vi "tiaoshi.vi"   [LabVIEW 2020]
types:
  T1 = enum32{"Invalid", "Standard", "Closed", "Hidden", "Minimized", "Maximized"}
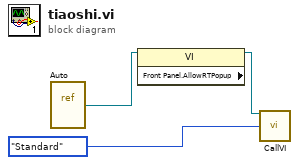
[diagram p0: block diagram]
diagram:
  n1 = vi-ref "Auto.vi"() -> (w2:refnum<vi>)
  n2 = property class="VI" props=["Front Panel.AllowRTPopup"](reference=w2) -> (reference out=w1:refnum<vi>)  [unwired: 1 in, 2 out]
  n3 = call "CallVI.vi"("VI引用"=w1, "状态"=T1."Standard") -> ()  [unwired: 12 in, 2 out]
